vi "to_json.vi"(8 "error in":errorcluster, 11 "ts.relative in":refnum<class "ts.relative.lvclass">) -> (0 "error out":errorcluster, 2 "json":string, 3 "ts.relative out":refnum<class "ts.relative.lvclass">)   [LabVIEW 2020, in "ts.relative.lvclass"]
uses:
  ts.relative.lvclass
  ts.relative.lvclass/ts.relative.ctl
  ac553a3d-6aa5-49ef-9e1c-caec14b63934.vi
  51cf98f5-1973-4989-a3e0-4cf140f0eb2f.vi
  <vilib>/LabVIEW Open Source Project/Epoch Date & Time/formatter.iso8601/Timestamp to ISO8601 UTC DateTime.vi
  <vilib>/JDP Science/JSONtext/Variant to JSON Text.vi
  <vilib>/JDP Science/JSONtext/LVClass Serializer/JSONtext LVClass Serializer.lvclass
  Nominal Client/Nominal Client.lvclass
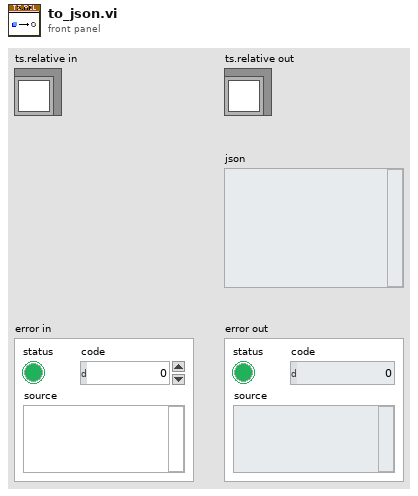
[diagram p1: front panel]
types:
  T1 = enum16{"DAYS", "HOURS", "MINUTES", "SECONDS", "MILLISECONDS", "MICROSECONDS", "NANOSECONDS", "PICOSECONDS"}
  T2 = cluster{"type":string, "relative":cluster{"timeUnit":string, "offset":string}}
  T3 = cluster{"type":string, "relative":cluster{"timeUnit":string}}
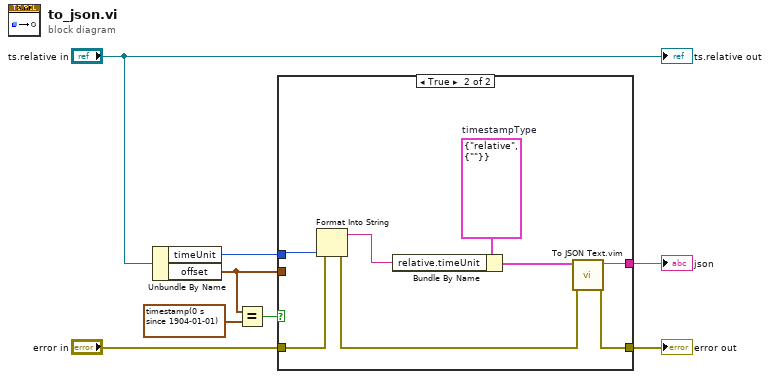
[diagram p0: block diagram]
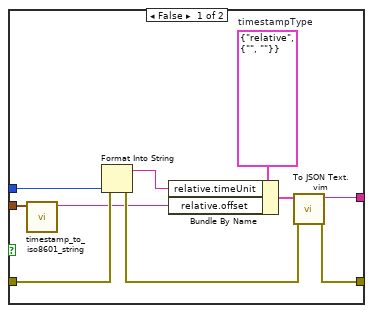
[diagram p2: hidden frame]
diagram:
  n1 = Unbundle By Name("ts.relative in") -> ("timeUnit"=w7:T1, "offset"=w6:timestamp)
  n2 = Equal?(x=w6, y=timestamp(0 s since 1904-01-01)) -> (x = y?=w4:bool)
  n3 = case shown="True" w4 {
    tunnel: w7 -> [w17 w23]
    tunnel: w6 -> [w18 _]
    tunnel: [w13 w22] -> w3
    tunnel: "error in" -> [w12 w21]
    tunnel: [w10 w19] -> w1
    frame False {
      w16 = T2 {"type"="relative", "relative"={"timeUnit"="", "offset"=""}}  # timestampType
      n4 = call "timestamp_to_iso8601_string.vi"("Time Stamp (now)"=w18) -> ("ISO8601 UTC DateTime"=w9:string)  [unwired: 10 in]
      n5 = Format Into String(error in=w12, w17) -> (resulting string=w15:string, error out=w11:errorcluster)  [unwired: 2 in]
      n6 = Bundle By Name(cluster=w16, "relative.timeUnit"=w15, "relative.offset"=w9) -> (w14:T2)
      n7 = call "To JSON Text.vim"("error in (no error)"=w11, "Anything"=w14) -> ("error out"=w10:errorcluster, "<JSON>"=w13:string)  [unwired: 8 in]
    }
    frame True {
      w26 = T3 {"type"="relative", "relative"={"timeUnit"=""}}  # timestampType
      n8 = Format Into String(error in=w21, w23) -> (resulting string=w25:string, error out=w20:errorcluster)  [unwired: 2 in]
      n9 = Bundle By Name(cluster=w26, "relative.timeUnit"=w25) -> (w24:T3)
      n10 = call "To JSON Text.vim"("error in (no error)"=w20, "Anything"=w24) -> ("error out"=w19:errorcluster, "<JSON>"=w22:string)  [unwired: 8 in]
    }
  }
  "error out" <- w1
  "json" <- w3
  "ts.relative out" <- "ts.relative in"
